vi "Photon-STR18_1_1.vi"() -> ()   [LabVIEW 2015]
uses:
  Menu.ctl
  <vilib>/Utility/file.llb/Write Delimited Spreadsheet (DBL).vi
panel:
  out "sizeA":i32
  out "mean 2":ext format="%0.2f"
  out "max index(es)":i32
  out "max value":u16
  out "Waveform Graph 5":dbl[][](graph)
  out "Waveform Graph 4":u8[][](graph)
  out "Size B":i32
  out "Size A":i32
  out "Waveform Graph 3":sgl[][](graph)
  out "8bits?":bool
  out "Waveform Graph 2":dbl[][](graph)
  out "P 2":i32=64
  out "m 2":i32=2
  in  "P":i32=64
  out "Numeric":i32
  out "sum A":dbl format="%#_10g"
  out "sum B":dbl format="%#_10g"
  out "Correlacion":cluster{ext[], ext[]}(graph)
  out "# of Channels":i32
  out "Duration":sgl
  in  "m":i32=2
  out "time":ext[](array[numeric])
  out "corr":ext[](array[numeric])
  out "d*(k)":dbl[][](array[numeric])
  out "Structura":cluster{ext[], ext[]}(graph)
  out "g(k) lineal":ext[](array[numeric])
  out "millisecond timer value":u32
  in  "Sample  time (a.u.)":sgl=1000.0
  out "segmentation ChA":sgl[](array[numeric])
  out "tau":dbl[](array[numeric]) format="%#_12g"
  out "Duration A [s]":dbl
  out "tau 3":dbl[](array[numeric]) format="%#_10g"
  out "Segmentation ChB 2":sgl[](array[numeric])
  out "Duration B [s] 2":dbl
  out "tamaño B 2":i32
  out "tau 2":dbl[](array[numeric]) format="%#_10g"
  out "Segmentation ChB":sgl[](array[numeric])
  out "Duration B [s]":dbl
  out "Size B":i32
  out "mean":dbl format="%0.2f"
  out "Size A":i32
  out "size(s) 2":i32
  out "time out":dbl[](array[numeric]) format="%#_10g"
  out "Max photon CHA 3":i32
  out "Numeric 2":i32
  out "size(s)":i32
  out "size(s) 7":i32
  out "Max photon CHA 4":i32
  out "size(s) 4":i32
  out "Max photon CHA 6":i32
  out "Numeric 3":i32
  out "size(s) 5":i32
  out "size(s) 6":i32
  out "Max photon CHA":i32
  out "Max photon CHA 2":i32
  out "element":sgl
  out "CHA":u8[](array[numeric])
  out "CHB":u8[](array[numeric])
  in  "Save Data":bool
  in  "Half data":bool
  in  "EXIT":bool
  in  "Open File":bool
  in  "Analysis":u16(ring) items=["Auto correlation A", "Auto correlation B", "Cross correlation AxB", "Cross correlation BxA"]
  in  "Data type":u16(ring) items=["Ascii", "Binary"]
  out "elapsed time in min":dbl
  out "Elapsed time (s)":dbl
  # "PhotonSTR-18"
  # "Parameters"
  # "Duration A"
  # "Total # of photons A"
  # "Channel A"
  # "Duration B"
  # "Total # of photons B"
  # "Operation Mode"
  # "Channel B"
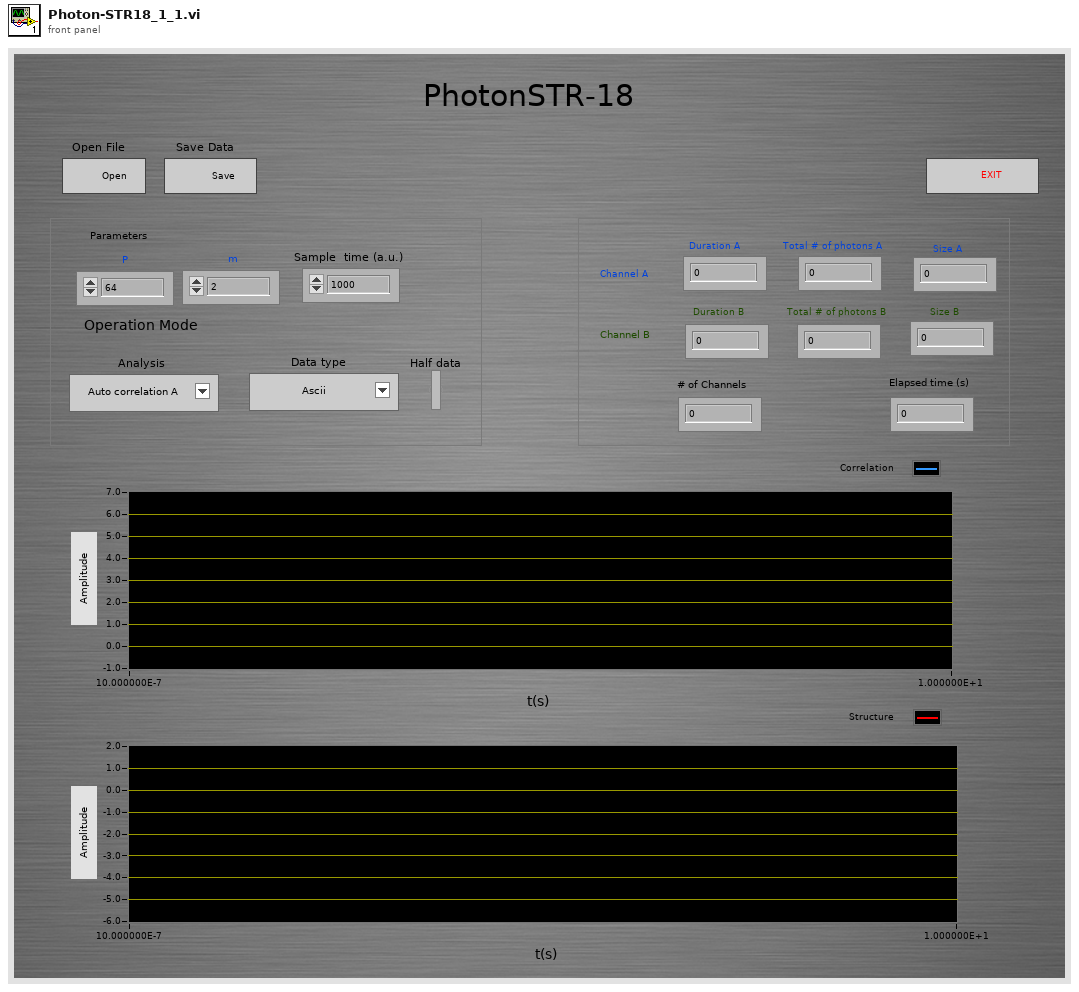
[diagram p1: front panel]
types:
  T1 = typedef "Menu.ctl" = enum16{"Init", "user action", "Load file", "Select range", "Process Photons(t)", "Process Segmentation", "Process Correlation ", "Save data", "Stop"}
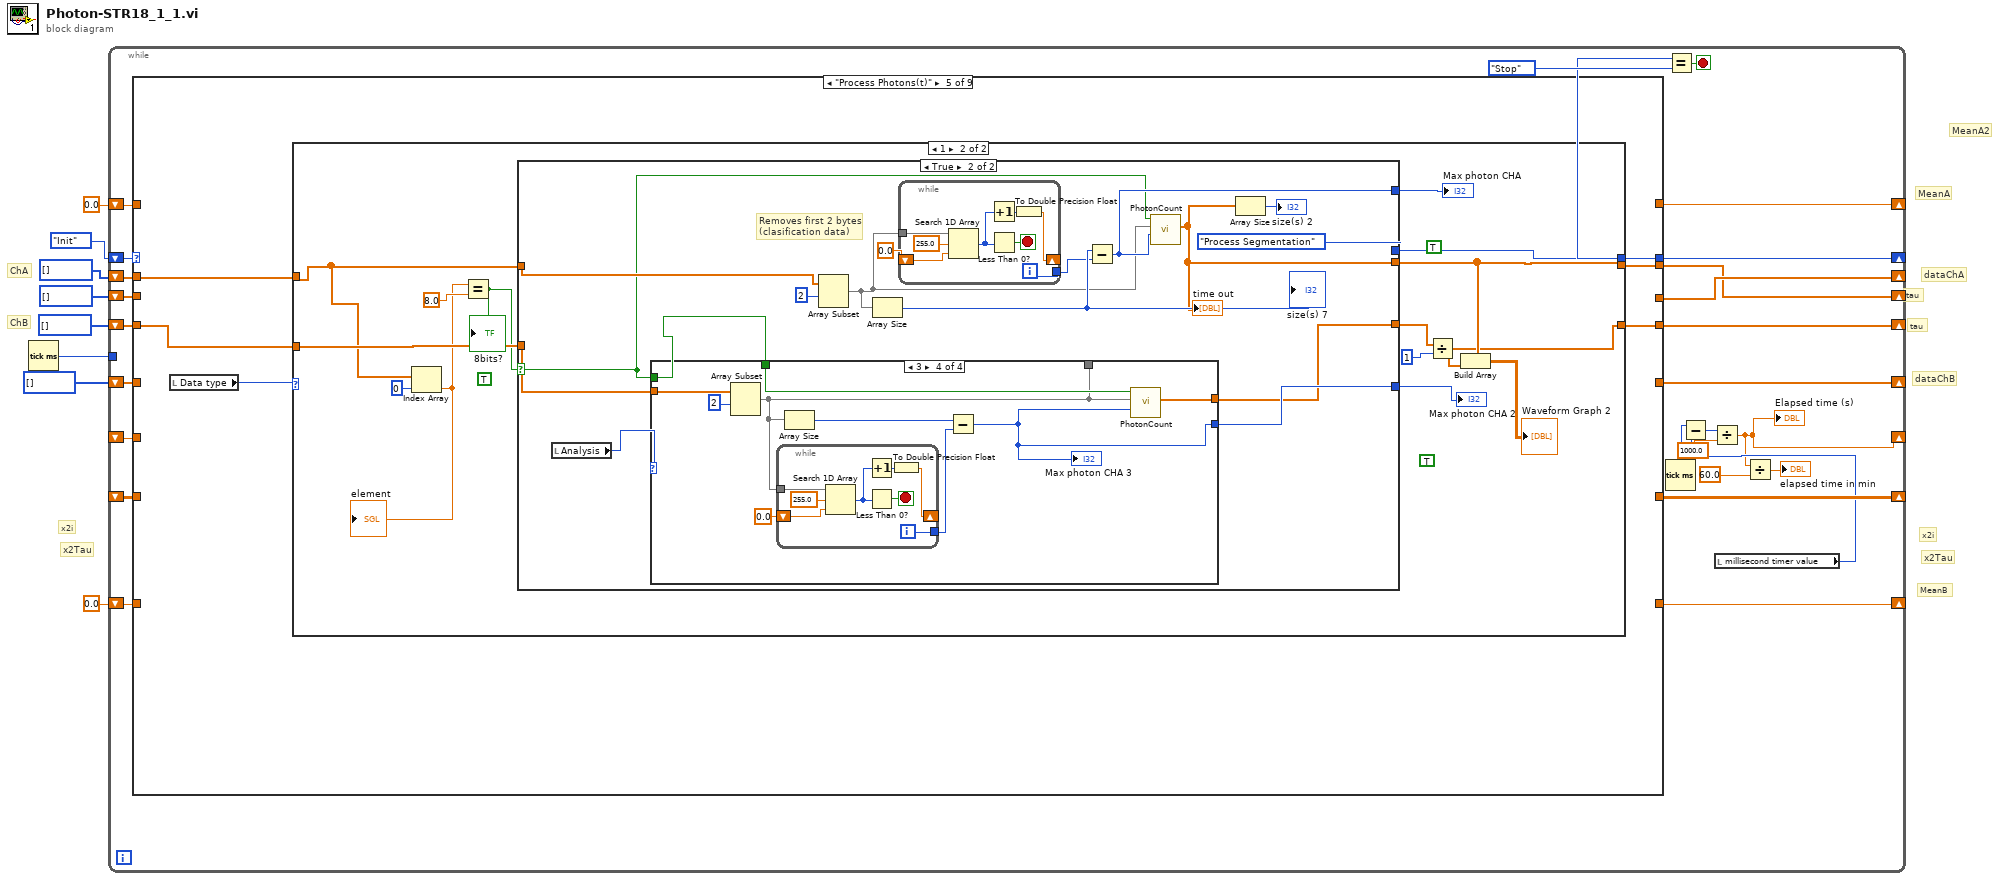
[diagram p0: block diagram]
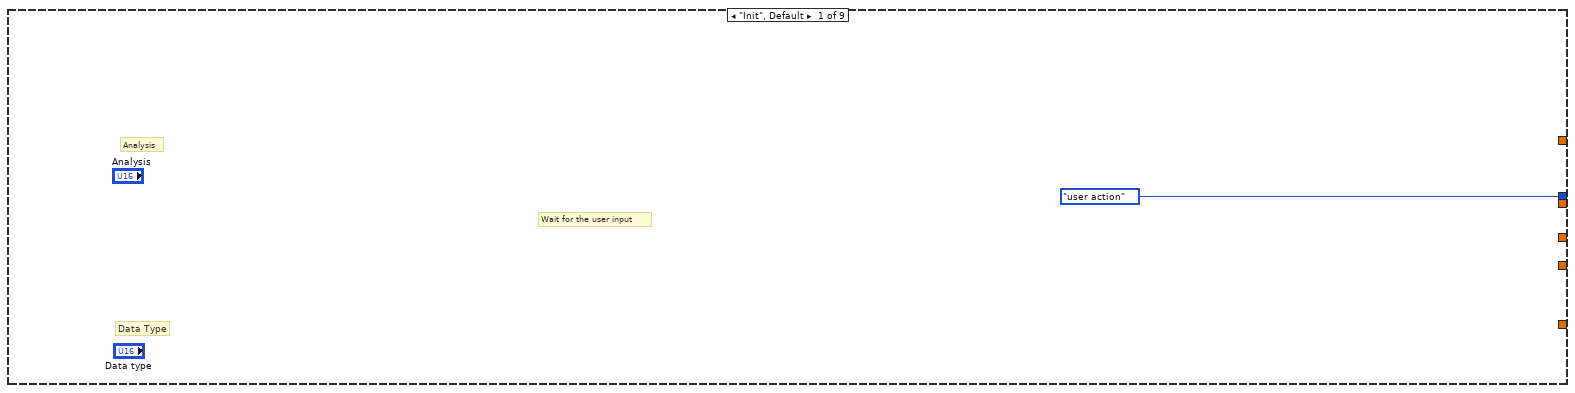
[diagram p2: hidden frame]
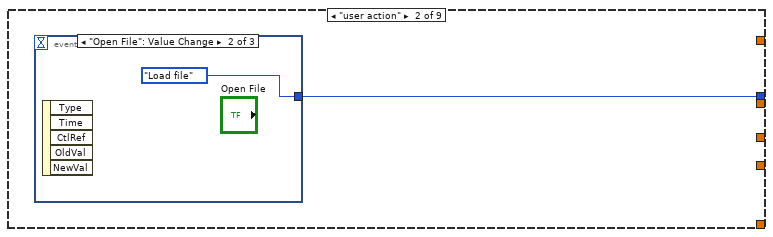
[diagram p3: hidden frame]
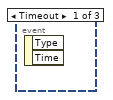
[diagram p4: hidden frame]
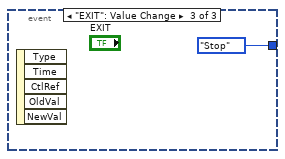
[diagram p5: hidden frame]
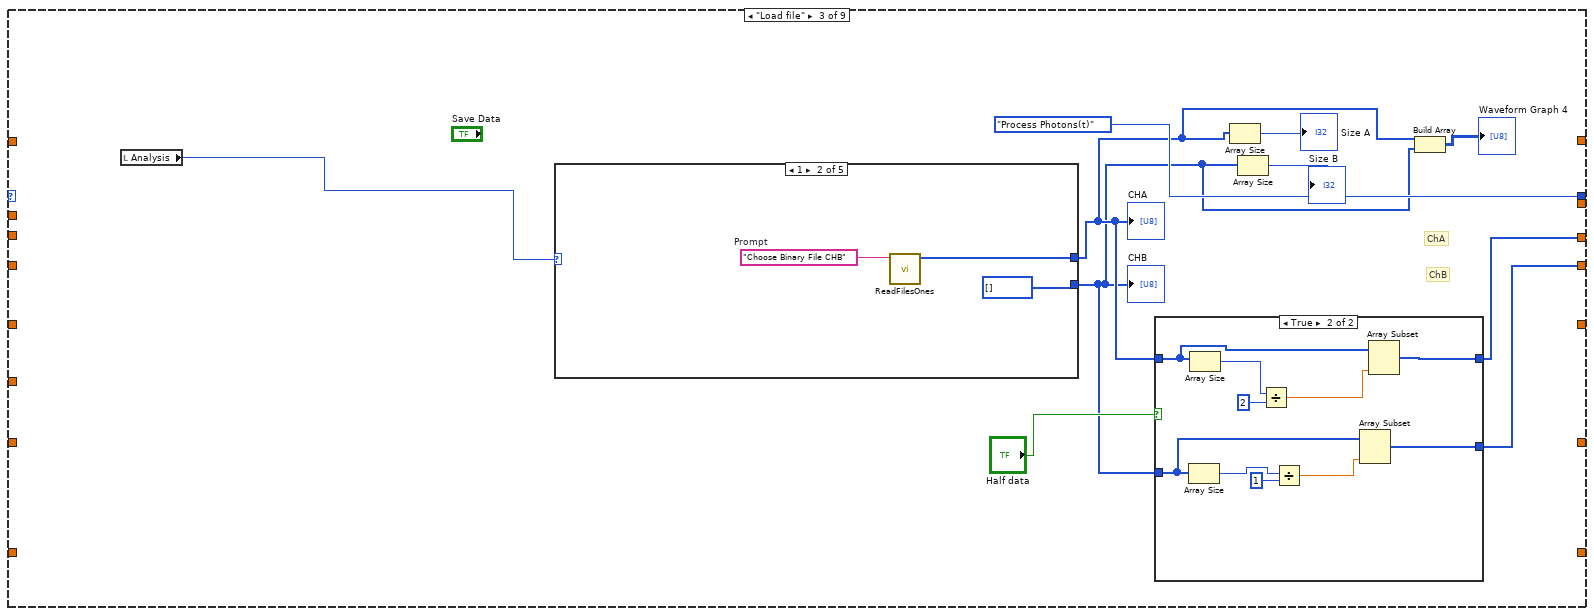
[diagram p6: hidden frame]
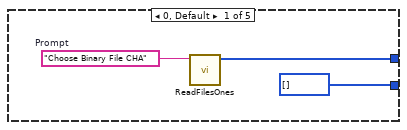
[diagram p8: hidden frame]
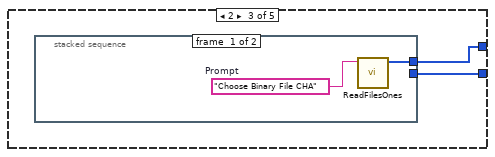
[diagram p9: hidden frame]
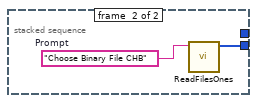
[diagram p10: hidden frame]
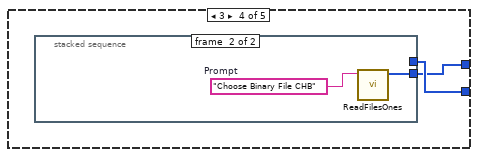
[diagram p11: hidden frame]
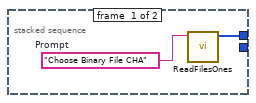
[diagram p12: hidden frame]
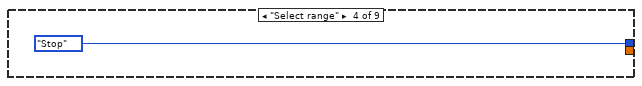
[diagram p14: hidden frame]
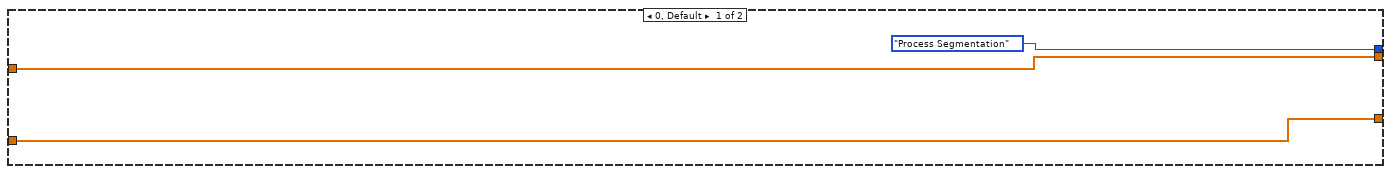
[diagram p15: hidden frame]
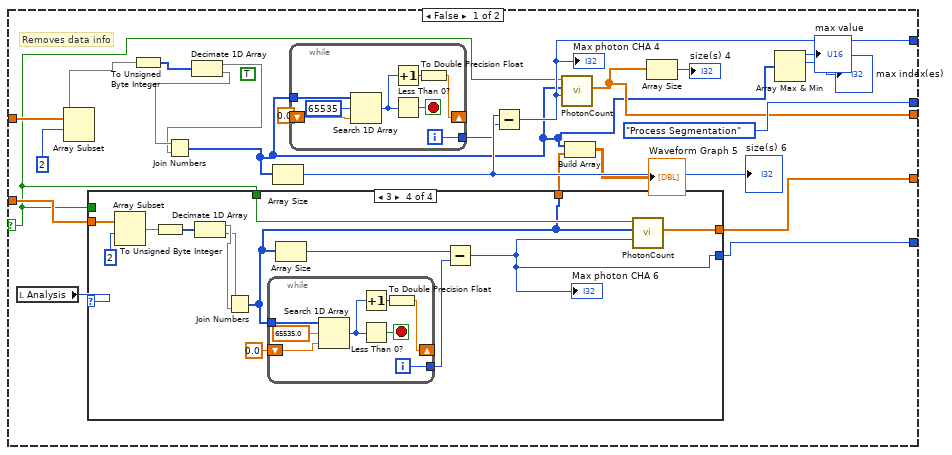
[diagram p16: hidden frame]
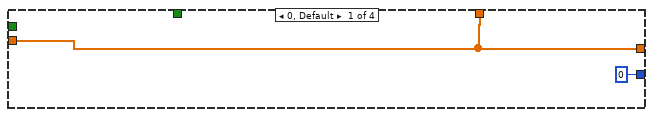
[diagram p17: hidden frame]
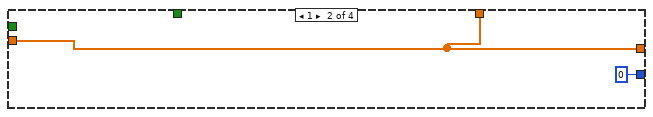
[diagram p18: hidden frame]
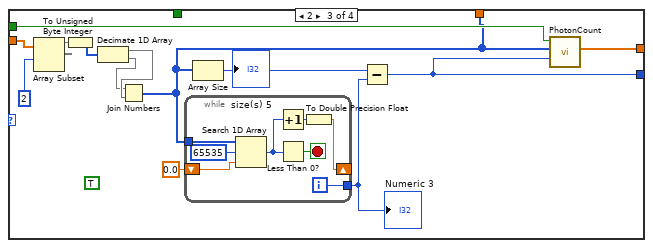
[diagram p19: hidden frame]
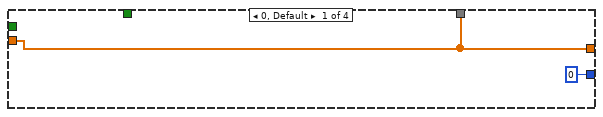
[diagram p20: hidden frame]
diagram:
  # "x2Tau"
  # "x2i"
  # "x2Tau"
  # "x2i"
  # "MeanA2"
  # "MeanB"
  # "MeanA"
  # "tau"
  # "tau"
  # "ChB"
  # "dataChB"
  # "dataChA"
  # "ChA"
  n1 = Tick Count (ms)() -> (millisecond timer value=w5:u32)
  n2 = while {
    shift-right: [w32] -> _
    shift-left: Menu."Init" ("Menu") -> [w34]
    shift-right: [w30] -> _
    shift-left: u32[] [] ("Photon trace A") -> [w29]
    shift-right: [w28] -> _
    shift-left: u32[] [] ("Photon trace A") -> [w27]
    shift-right: [w16] -> _
    shift-left: _ -> [w26]
    tunnel: w5 -> [_]
    shift-right: [w20] -> _
    shift-left: u32[] [] ("Photon trace A") -> [w19]
    shift-right: [w18] -> _
    shift-left: u32[] [] ("Photon trace A") -> [w17]
    shift-right: [w13] -> _
    shift-left: _ -> [w15]
    shift-right: [w12] -> _
    shift-left: 0.0 ("mean") -> [w10]
    shift-right: [w11] -> _
    shift-left: 0.0 ("mean") -> [w9]
    stop <- w31 stop-if-true
    n3 = case shown="\"Process Photons(t)\"" w34 {
      tunnel: [Menu."user action" ("Menu") w36 Menu."Process Photons(t)" ("Menu") Menu."Stop" ("Menu") w85 Menu."Process Correlation " ("Menu") Menu."Save data" ("Menu") Menu."Stop" ("Menu") Menu."Stop" ("Menu")] -> w32
      tunnel: [_ _ w44 _ _ w244 _ _ _] -> w30
      tunnel: w29 -> [_ _ _ _ w84 _ w336 _ _]
      tunnel: [_ _ _ _ w81 w252 _ _ _] -> w28
      tunnel: w27 -> [_ _ _ _ _ w261 w340 _ _]
      tunnel: [_ _ _ _ _ _ w369 _ _] -> w16
      tunnel: w26 -> [_ _ _ _ _ _ _ w435 _]
      tunnel: [_ _ w45 _ w82 w250 _ _ _] -> w20
      tunnel: w19 -> [_ _ _ _ w83 w262 _ _ _]
      tunnel: [_ _ _ _ _ w246 _ _ _] -> w18
      tunnel: w17 -> [_ _ _ _ _ _ w335 _ _]
      tunnel: w15 -> [_ _ _ _ _ _ _ _ _]
      tunnel: [_ _ _ _ _ w241 _ _ _] -> w12
      tunnel: [_ _ _ _ _ w248 _ _ _] -> w11
      tunnel: w10 -> [_ _ _ _ _ _ w368 _ _]
      tunnel: w9 -> [_ _ _ _ _ _ w367 _ _]
      frame "Init", Default {
        # "Data Type"
        # "Analysis"
        # "Wait for the user input"
      }
      frame "user action" {
        n4 = event shown="[1] \"Open File\": Value Change" {
          selector: _ -> [_ _ _]
          dyn-events: _ -> [_ _ _]
          timeout: _ -> [_ _ _]
          tunnel: [_ Menu."Load file" ("Menu") Menu."Stop" ("Menu")] -> w36
          event Timeout {
            n5 = event-data() -> ()  [unwired: 1 in, 2 out]
          }
          event "Open File": Value Change {
            n6 = event-data() -> ()  [unwired: 1 in, 5 out]
          }
          event "EXIT": Value Change {
            n7 = event-data() -> ()  [unwired: 1 in, 5 out]
          }
        }
      }
      frame "Load file" {
        # "ChB"
        # "ChA"
        n8 = local read "Analysis"() -> (w47:u16)
        n9 = case shown="1" w47 {
          tunnel: [w62 w65 w68 w73 _] -> w41
          tunnel: [u8[] [] u8[] [] w67 w74 _] -> w40
          frame 0, Default {
            w63 = "Choose Binary File CHA"  # Prompt
            n10 = call "ReadFilesOnes.vi"("prompt"=w63) -> ("Data"=w62:u8[])  [unwired: 8 in, 2 out]
          }
          frame 1 {
            w66 = "Choose Binary File CHB"  # Prompt
            n11 = call "ReadFilesOnes.vi"("prompt"=w66) -> ("Data"=w65:u8[])  [unwired: 8 in, 2 out]
          }
          frame 2 {
            n12 = stacked-sequence {
              tunnel: [w69 _] -> w68
              tunnel: [_ w71] -> w67
              frame #0 {
                w70 = "Choose Binary File CHA"  # Prompt
                n13 = call "ReadFilesOnes.vi"("prompt"=w70) -> ("Data"=w69:u8[])  [unwired: 8 in, 2 out]
              }
              frame #1 {
                w72 = "Choose Binary File CHB"  # Prompt
                n14 = call "ReadFilesOnes.vi"("prompt"=w72) -> ("Data"=w71:u8[])  [unwired: 8 in, 2 out]
              }
            }
          }
          frame 3 {
            n15 = stacked-sequence {
              tunnel: [w75 _] -> w74
              tunnel: [_ w77] -> w73
              frame #0 {
                w76 = "Choose Binary File CHA"  # Prompt
                n16 = call "ReadFilesOnes.vi"("prompt"=w76) -> ("Data"=w75:u8[])  [unwired: 8 in, 2 out]
              }
              frame #1 {
                w78 = "Choose Binary File CHB"  # Prompt
                n17 = call "ReadFilesOnes.vi"("prompt"=w78) -> ("Data"=w77:u8[])  [unwired: 8 in, 2 out]
              }
            }
          }
          frame 4 {
          }
        }
        "CHA" <- w41
        "CHB" <- w40
        n18 = case shown="True" "Half data" {
          tunnel: w41 -> [w50 w60]
          tunnel: w40 -> [w49 w59]
          tunnel: [w50 w57] -> w44
          tunnel: [w49 w56] -> w45
          frame False {
          }
          frame True {
            n19 = Array Size(array=w59) -> (size(s)=w55:i32)
            n20 = Array Size(array=w60) -> (size(s)=w58:i32)
            n21 = Divide(x=w58, y=2) -> (x/y=w54:dbl)
            n22 = Divide(x=w55, y=1) -> (x/y=w53:dbl)
            n23 = Array Subset(array=w59, length=w53) -> (w56:u8[])  [unwired: 1 in]
            n24 = Array Subset(array=w60, length=w54) -> (w57:u8[])  [unwired: 1 in]
          }
        }
        n25 = Array Size(array=w41) -> (size(s)=→"Size A":i32)
        n26 = Array Size(array=w40) -> (size(s)=→"Size B":i32)
        n27 = Build Array(w41, w40) -> (→"Waveform Graph 4":u8[][])
      }
      frame "Select range" {
      }
      frame "Process Photons(t)" {
        n28 = local read "Data type"() -> (w80:u16)
        n29 = case shown="1" w80 {
          tunnel: [Menu."Process Segmentation" ("Menu") w101] -> w85
          tunnel: w84 -> [w87 w99]
          tunnel: w83 -> [w86 w102]
          tunnel: [w86 w89] -> w82
          tunnel: [w87 w93] -> w81
          frame 0, Default {
          }
          frame 1 {
            (unwired) TRUE ("transpose? (no:F)")
            (unwired) TRUE ("transpose? (no:F)")
            (unwired) TRUE
            n30 = Index Array(array=w99, index=0) -> (element=w97:sgl)
            "element" <- w97
            n31 = Equal?(x=w97, y=8.0) -> (x = y?=w94:bool)
            "8bits?" <- w94
            n32 = case shown="True" w94 {
              selector: w94 -> [w103 w181]
              tunnel: w102 -> [w115 w189]
              tunnel: [w120 w182] -> w91
              tunnel: [w116 w188] -> w93
              tunnel: [Menu."Process Segmentation" ("Menu") Menu."Process Segmentation" ("Menu")] -> w101
              tunnel: w99 -> [w113 w185]
              tunnel: [w117 w184] -> w96
              tunnel: [w118 w183] -> w95
              frame False {
                (unwired) TRUE ("transpose? (no:F)")
                # "Removes data info"
                n33 = local read "Analysis"() -> (w119:u16)
                n34 = Array Subset(array=w113, index=2) -> (w105:sgl[])  [unwired: 1 in]
                n35 = case shown="3" w119 {
                  tunnel: w115 -> [w126 w128 w135 w156]
                  tunnel: [w126 w128 w138 w159] -> w120
                  tunnel: [0 0 w137 w158] -> w118
                  tunnel: w103 -> [_ _ w136 _]
                  tunnel: w103 -> [_ _ _ w157]
                  tunnel: [w126 w128 w132 w153] -> w110
                  frame 0, Default {
                  }
                  frame 1 {
                  }
                  frame 2 {
                    (unwired) TRUE ("transpose? (no:F)")
                    n36 = Array Subset(array=w135, index=2) -> (w131:dbl[])  [unwired: 1 in]
                    n37 = To Unsigned Byte Integer(number=w131) -> (unsigned 8bit integer=w130:u8[])
                    n38 = Decimate 1D Array(w130) -> (w134:u8[], w133:u8[])
                    n39 = Join Numbers(hi=w133, lo=w134) -> ((hi.lo)=w132:u16[])
                    n40 = while {
                      tunnel: w132 -> [w150]
                      shift-right: [w143] -> _
                      shift-left: 0.0 ("element") -> [w148]
                      tunnel: [w146] -> w139
                      i -> [w146]
                      stop <- w147 stop-if-true
                      n41 = Search 1D Array(1D array=w150, element=u16 65535, start index (0)=w148) -> (index of element=w145:i32)
                      n42 = Increment(x=w145) -> (x+1=w144:i32)
                      n43 = Less Than 0?(x=w145) -> (x < 0?=w147:bool)
                      n44 = To Double Precision Float(number=w144) -> (double precision float=w143:dbl)
                    }
                    "Numeric 3" <- w139
                    n45 = Array Size(array=w132) -> (size(s)=w140:i32)
                    "size(s) 5" <- w140
                    n46 = Subtract(x=w140, y=w139) -> (x-y=w137:i32)
                    n47 = call "PhotonCount.vi"("# Photons"=w137, "Data in"=w132, "Boolean"=w136) -> ("time out"=w138:dbl[])  [unwired: 8 in]
                  }
                  frame 3 {
                    n48 = Array Subset(array=w156, index=2) -> (w152:dbl[])  [unwired: 1 in]
                    n49 = To Unsigned Byte Integer(number=w152) -> (unsigned 8bit integer=w151:u8[])
                    n50 = Decimate 1D Array(w151) -> (w155:u8[], w154:u8[])
                    n51 = Join Numbers(hi=w154, lo=w155) -> ((hi.lo)=w153:u16[])
                    n52 = while {
                      tunnel: w153 -> [w171]
                      shift-right: [w164] -> _
                      shift-left: 0.0 ("element") -> [w169]
                      tunnel: [w167] -> w160
                      i -> [w167]
                      stop <- w168 stop-if-true
                      n53 = Search 1D Array(1D array=w171, element=sgl 65535.0, start index (0)=w169) -> (index of element=w166:i32)
                      n54 = Increment(x=w166) -> (x+1=w165:i32)
                      n55 = Less Than 0?(x=w166) -> (x < 0?=w168:bool)
                      n56 = To Double Precision Float(number=w165) -> (double precision float=w164:dbl)
                    }
                    n57 = Array Size(array=w153) -> (size(s)=w161:i32)
                    n58 = Subtract(x=w161, y=w160) -> (x-y=w158:i32)
                    "Max photon CHA 6" <- w158
                    n59 = call "PhotonCount.vi"("# Photons"=w158, "Data in"=w153, "Boolean"=w157) -> ("time out"=w159:dbl[])  [unwired: 8 in]
                  }
                }
                n60 = To Unsigned Byte Integer(number=w105) -> (unsigned 8bit integer=w104:u8[])
                n61 = Decimate 1D Array(w104) -> (w111:u8[], w112:u8[])
                n62 = Join Numbers(hi=w112, lo=w111) -> ((hi.lo)=w108:u16[])
                n63 = Array Size(array=w108) -> (size(s)=w124:i32)
                "size(s) 6" <- w124
                n64 = while {
                  tunnel: w108 -> [w179]
                  shift-right: [w173] -> _
                  shift-left: 0.0 ("element") -> [w177]
                  tunnel: [w172] -> w123
                  i -> [w172]
                  stop <- w176 stop-if-true
                  n65 = Search 1D Array(1D array=w179, element=u16 65535, start index (0)=w177) -> (index of element=w175:i32)
                  n66 = Increment(x=w175) -> (x+1=w174:i32)
                  n67 = Less Than 0?(x=w175) -> (x < 0?=w176:bool)
                  n68 = To Double Precision Float(number=w174) -> (double precision float=w173:dbl)
                }
                n69 = Subtract(x=w124, y=w123) -> (x-y=w117:i32)
                "Max photon CHA 4" <- w117
                n70 = call "PhotonCount.vi"("# Photons"=w117, "Data in"=w108, "Boolean"=w103) -> ("time out"=w116:dbl[])  [unwired: 8 in]
                n71 = Build Array(w108, w110) -> (→"Waveform Graph 5":dbl[][])
                n72 = Array Size(array=w116) -> (size(s)=→"size(s) 4":i32)
                n73 = Array Max & Min(array=w108) -> (max value=→"max value":u16, max index (indices)=→"max index(es)":i32)  [unwired: 2 out]
              }
              frame True {
                # "Removes first 2 bytes\n(clasification data)"
                n74 = local read "Analysis"() -> (w186:u16)
                n75 = case shown="3" w186 {
                  tunnel: w189 -> [w195 w197 w206 w220]
                  tunnel: [w195 w197 w202 w219] -> w182
                  tunnel: [0 0 w201 w218] -> w183
                  tunnel: w181 -> [_ _ w200 _]
                  tunnel: w181 -> [_ _ _ w217]
                  tunnel: [w195 w197 w199 w216] -> _
                  frame 0, Default {
                  }
                  frame 1 {
                  }
                  frame 2 {
                    n76 = Array Subset(array=w206, index=2) -> (w199:dbl[])  [unwired: 1 in]
                    n77 = while {
                      tunnel: w199 -> [w215]
                      shift-right: [w208] -> _
                      shift-left: 0.0 ("element") -> [w213]
                      tunnel: [w211] -> w203
                      i -> [w211]
                      stop <- w212 stop-if-true
                      n78 = Search 1D Array(1D array=w215, element=sgl 255.0, start index (0)=w213) -> (index of element=w210:i32)
                      n79 = Increment(x=w210) -> (x+1=w209:i32)
                      n80 = Less Than 0?(x=w210) -> (x < 0?=w212:bool)
                      n81 = To Double Precision Float(number=w209) -> (double precision float=w208:dbl)
                    }
                    "Numeric 2" <- w203
                    n82 = Array Size(array=w199) -> (size(s)=w204:i32)
                    "size(s)" <- w204
                    n83 = Subtract(x=w204, y=w203) -> (x-y=w201:i32)
                    n84 = call "PhotonCount.vi"("# Photons"=w201, "Data in"=w199, "Boolean"=w200) -> ("time out"=w202:dbl[])  [unwired: 8 in]
                  }
                  frame 3 {
                    n85 = Array Subset(array=w220, index=2) -> (w216:dbl[])  [unwired: 1 in]
                    n86 = while {
                      tunnel: w216 -> [w232]
                      shift-right: [w225] -> _
                      shift-left: 0.0 ("element") -> [w230]
                      tunnel: [w228] -> w221
                      i -> [w228]
                      stop <- w229 stop-if-true
                      n87 = Search 1D Array(1D array=w232, element=sgl 255.0, start index (0)=w230) -> (index of element=w227:i32)
                      n88 = Increment(x=w227) -> (x+1=w226:i32)
                      n89 = Less Than 0?(x=w227) -> (x < 0?=w229:bool)
                      n90 = To Double Precision Float(number=w226) -> (double precision float=w225:dbl)
                    }
                    n91 = Array Size(array=w216) -> (size(s)=w222:i32)
                    n92 = Subtract(x=w222, y=w221) -> (x-y=w218:i32)
                    "Max photon CHA 3" <- w218
                    n93 = call "PhotonCount.vi"("# Photons"=w218, "Data in"=w216, "Boolean"=w217) -> ("time out"=w219:dbl[])  [unwired: 8 in]
                  }
                }
                n94 = Array Subset(array=w185, index=2) -> (w180:sgl[])  [unwired: 1 in]
                n95 = Array Size(array=w180) -> (size(s)=w192:i32)
                "size(s) 7" <- w192
                n96 = while {
                  tunnel: w180 -> [w240]
                  shift-right: [w233] -> _
                  shift-left: 0.0 ("element") -> [w238]
                  tunnel: [w236] -> w191
                  i -> [w236]
                  stop <- w237 stop-if-true
                  n97 = Search 1D Array(1D array=w240, element=sgl 255.0, start index (0)=w238) -> (index of element=w235:i32)
                  n98 = Increment(x=w235) -> (x+1=w234:i32)
                  n99 = Less Than 0?(x=w235) -> (x < 0?=w237:bool)
                  n100 = To Double Precision Float(number=w234) -> (double precision float=w233:dbl)
                }
                n101 = Subtract(x=w192, y=w191) -> (x-y=w184:i32)
                n102 = call "PhotonCount.vi"("# Photons"=w184, "Data in"=w180, "Boolean"=w181) -> ("time out"=w188:dbl[])  [unwired: 8 in]
                "time out" <- w188
                n103 = Array Size(array=w188) -> (size(s)=→"size(s) 2":i32)
              }
            }
            "Max photon CHA" <- w96
            "Max photon CHA 2" <- w95
            n104 = Divide(x=w91, y=1 ("Data Type (DBL)")) -> (x/y=w89:dbl[])
            n105 = Build Array(w93, w89) -> (→"Waveform Graph 2":dbl[][])
          }
        }
      }
      frame "Process Segmentation" {
        w255 = 60000000.0 ("x")
        # "Estima la segmentacion de datos"
        n106 = local read "Analysis"() -> (w245:u16)
        n107 = call "Segmentation.vi"("sample time"="Sample  time (a.u.)", "relative time"=w261) -> ("Segmentation"=w242:sgl[], "mean"=w241:dbl, "tau"=w243:dbl[])  [unwired: 7 in]
        "segmentation ChA" <- w242
        "tau" <- w243
        "mean 2" <- w241
        n108 = Array Size(array=w242) -> (size(s)=w247:i32)
        "Size A" <- w247
        "sizeA" <- w247
        n109 = case shown="2" w245 {
          tunnel: w262 -> [w268 w272 w284 w291]
          tunnel: "Sample  time (a.u.)" -> [_ _ w283 w290]
          tunnel: w255 -> [_ _ w278 w289]
          tunnel: [w266 w271 w276 w287] -> w253
          tunnel: [w268 w272 w277 w288] -> w251
          tunnel: [sgl[] [] sgl[] [] w274 w285] -> w249
          tunnel: w247 -> [w266 w271 _ _]
          tunnel: [0.0 ("mean") 0.0 ("mean") w275 w286] -> w248
          tunnel: w242 -> [w264 w269 _ _]
          tunnel: [w264 w269 w274 w285] -> _
          frame 0, Default {
          }
          frame 1 {
          }
          frame 2 {
            n110 = call "Segmentation.vi"("sample time"=w283, "relative time"=w284) -> ("Segmentation"=w274:sgl[], "mean"=w275:dbl, "tau"=w277:dbl[])  [unwired: 7 in]
            "tau 2" <- w277
            "Segmentation ChB" <- w274
            "mean" <- w275
            n111 = Array Size(array=w277) -> (size(s)=w276:i32)
            "Size B" <- w276
            n112 = Decrement(x=w276) -> (x-1=w282:i32)
            n113 = Index Array(array=w277, index=w282) -> (element=w281:dbl)
            n114 = Reciprocal(x=w278) -> (1/x=w280:dbl)
            n115 = Multiply(x=w281, y=w280) -> (x*y=→"Duration B [s]":dbl)
          }
          frame 3 {
            n116 = call "Segmentation.vi"("sample time"=w290, "relative time"=w291) -> ("Segmentation"=w285:sgl[], "mean"=w286:dbl, "tau"=w288:dbl[])  [unwired: 7 in]
            "tau 3" <- w288
            "Segmentation ChB 2" <- w285
            n117 = Array Size(array=w288) -> (size(s)=w287:i32)
            "tamaño B 2" <- w287
            n118 = Decrement(x=w287) -> (x-1=w295:i32)
            n119 = Index Array(array=w288, index=w295) -> (element=w294:dbl)
            n120 = Reciprocal(x=w289) -> (1/x=w293:dbl)
            n121 = Multiply(x=w294, y=w293) -> (x*y=→"Duration B [s] 2":dbl)
          }
        }
        n122 = Decrement(x=w247) -> (x-1=w259:i32)
        n123 = Index Array(array=w243, index=w259) -> (element=w256:dbl)
        n124 = Reciprocal(x=w255) -> (1/x=w258:dbl)
        n125 = Multiply(x=w256, y=w258) -> (x*y=→"Duration A [s]":dbl)
        n126 = Equal?(x=w247, y=w253) -> (x = y?=w254:bool)
        n127 = case shown="False" w254 {
          tunnel: w243 -> [w304 w324]
          tunnel: w242 -> [w303 w323]
          tunnel: w251 -> [w300 w326]
          tunnel: w249 -> [w301 w325]
          tunnel: w247 -> [w307 _]
          tunnel: w253 -> [w308 _]
          tunnel: [w299 w324] -> w252
          tunnel: [w298 w323] -> w244
          tunnel: [w297 w326] -> w250
          tunnel: [w296 w325] -> w246
          frame False {
            # "ChA>ChB"
            n128 = Greater?(x=w307, y=w308) -> (0:w305:bool)
            n129 = Subtract(x=w308, y=w307) -> (x-y=w306:i32)
            n130 = Absolute Value(x=w306) -> (abs(x)=w302:i32)
            n131 = case shown="False" w305 {
              tunnel: w304 -> [w310 w322]
              tunnel: w303 -> [w309 w321]
              tunnel: w302 -> [w315 w320]
              tunnel: [w310 w319] -> w299
              tunnel: [w309 w318] -> w298
              tunnel: w301 -> [w313 w316]
              tunnel: w300 -> [w314 w317]
              tunnel: [w311 w317] -> w297
              tunnel: [w312 w316] -> w296
              frame False {
                n132 = Delete From Array(array=w314, length=w315) -> (array with subset deleted=w311:dbl[])  [unwired: 1 in, 1 out]
                n133 = Delete From Array(array=w313, length=w315) -> (array with subset deleted=w312:sgl[])  [unwired: 1 in, 1 out]
              }
              frame True {
                n134 = Delete From Array(array=w322, length=w320) -> (array with subset deleted=w319:dbl[])  [unwired: 1 in, 1 out]
                n135 = Delete From Array(array=w321, length=w320) -> (array with subset deleted=w318:sgl[])  [unwired: 1 in, 1 out]
              }
            }
          }
          frame True {
          }
        }
      }
      frame "Process Correlation " {
        (unwired) 1.0 ("y")
        # "Calcula correlacion"
        # "g(k)=[G(k)-n0AnkB]/(n0AnkB))"
        # "Normalize"
        # "Compara que el tamaño\nde segmentation sea multiplo de m"
        n136 = Divide(x=w335, y=2 ("lower limit")) -> (x/y=w343:sgl[])
        n137 = Build Array(w336, w343) -> (→"Waveform Graph 3":sgl[][])
        n138 = To Double Precision Float(number=w335) -> (double precision float=w356:dbl[])
        n139 = To Double Precision Float(number=w336) -> (double precision float=w357:dbl[])
        n140 = while {
          tunnel: [w397] -> w328 mode=indexing
          shift-right: [w393] -> _
          shift-left: w357 -> [w390]
          tunnel: "m" -> [w387]
          tunnel: "P" -> [w388]
          tunnel: [w395] -> w337 mode=indexing
          shift-right: [w382] -> _
          shift-left: w356 -> [w389]
          tunnel: w368 -> [w386]
          tunnel: w367 -> [w385]
          tunnel: [w384] -> w331
          tunnel: [w383] -> w334
          tunnel: [w381] -> w327
          i -> [w394]
          stop <- w398 stop-if-true
          n141 = local read "Analysis"() -> (w381:u16)
          n142 = case shown="1" w381 {
            tunnel: w390 -> [w424 w426 w430 w434]
            tunnel: [w424 w426 w430 w434] -> w380
            tunnel: [w424 w426 w429 w433] -> w379
            tunnel: w389 -> [_ _ w429 w433]
            tunnel: w386 -> [w423 w425 w428 w432]
            tunnel: w385 -> [_ _ w427 w431]
            tunnel: [w423 w425 w428 w432] -> w384
            tunnel: [w423 w425 w427 w431] -> w383
            frame 0, Default {
            }
            frame 1 {
            }
            frame 2 {
            }
            frame 3 {
            }
          }
          n143 = case shown="0, Default" w381 {
            tunnel: [w403 w408 w415 w422] -> w397
            tunnel: w388 -> [w401 w406 w414 w417]
            tunnel: w387 -> [w400 w405 w413 w416]
            tunnel: [w399 w404 w412 w421] -> w393
            tunnel: [w399 w404 w411 w420] -> w382
            tunnel: w379 -> [_ _ w410 w418]
            tunnel: w380 -> [w402 w407 w409 w419]
            frame 0, Default {
              n144 = call "Auto_corr.vi"("m"=w400, "P"=w401, "input A"=w402) -> ("Sn"=w399:dbl[], "Acc"=w403:dbl[])  [unwired: 7 in]
            }
            frame 1 {
              n145 = call "Auto_corr.vi"("m"=w405, "P"=w406, "input A"=w407) -> ("Sn"=w404:dbl[], "Acc"=w408:dbl[])  [unwired: 7 in]
            }
            frame 2 {
              n146 = call "Cross_corr.vi"("m"=w413, "P"=w414, "input B"=w410, "input A"=w409) -> ("Sn A"=w412:dbl[], "Acc"=w415:dbl[], "Sn B"=w411:dbl[])  [unwired: 5 in]
            }
            frame 3 {
              n147 = call "Cross_corr.vi"("m"=w416, "P"=w417, "input B"=w418, "input A"=w419) -> ("Sn A"=w421:dbl[], "Acc"=w422:dbl[], "Sn B"=w420:dbl[])  [unwired: 5 in]
            }
          }
          n148 = Array Size(array=w393) -> (size(s)=w396:i32)
          n149 = Add Array Elements(numeric array=w393) -> (sum=→"sum A":dbl)
          n150 = Add Array Elements(numeric array=w382) -> (sum=→"sum B":dbl)
          n151 = Less Or Equal?(x=w396, y=w387) -> (x <= y?=w398:bool)
          n152 = Array Size(array=w380) -> (size(s)=w395:i32)
          "Numeric" <- w394
        }
        n153 = call "Normalizer.vi"("Acc"=w328, "m"="m", "p"="P", "Tamaño Sn"=w337, "Analysis 2"=w327, "AvgA"=w331, "DataA"=w336, "AvgB"=w334, "DataB"=w335) -> ("g(k)"=w333:dbl[][], "s(k)"=w330:dbl[][])  [unwired: 9 in]
        "d*(k)" <- w330
        n154 = Array Size(array=w328) -> (size(s)=w329:i32[])
        n155 = call "Data_select.vi"("m"="m", "P"="P", "d(k) in"=w330, "g(k) in"=w333) -> ("d(k) lineal"=w352:ext[], "g(k) lineal"=w342:ext[])  [unwired: 6 in]
        "g(k) lineal" <- w342
        n156 = Tick Count (ms)() -> (millisecond timer value=→"millisecond timer value":u32)
        n157 = Index Array(array=w329, index=0) -> (element=w358:i32)
        n158 = case shown="True" TRUE {
          tunnel: w342 -> [w372 w374]
          tunnel: [w371 w373] -> w349
          frame False {
            n159 = Array Size(array=w372) -> (size(s)=w371:i32)
          }
          frame True {
            n160 = while {
              tunnel: w374 -> [w378] mode=indexing
              tunnel: [w375] -> w373
              i -> [w376]
              stop <- w377 stop-if-true
              n161 = Not A Number/Path/Refnum?(number/path/refnum=w378) -> (NaN/Path/Refnum?=w377:bool)
              n162 = To Double Precision Float(number=w376) -> (double precision float=w375:dbl)
            }
          }
        }
        n163 = call "multi-tau_time.vi"("tau"=w340, "m"="m", "P"="P", "No. of shift registers"=w358) -> ("time multi-tau"=w341:ext[])  [unwired: 7 in]
        n164 = Divide(x=w341, y=60000000.0) -> (x/y=w332:ext[])
        n165 = Array Subset(array=w352, index=0) -> (w348:ext[])  [unwired: 1 in]
        n166 = Array Subset(array=w342, index=0, length=w349) -> (w355:ext[])
        "corr" <- w355
        n167 = Array Subset(array=w332, index=0, length=w349) -> (w350:ext[])
        "time" <- w350
        n168 = Array Size(array=w355) -> (size(s)=→"# of Channels":i32)
        n169 = Bundle(w350, w355) -> (→"Correlacion":cluster{ext[], ext[]})  [unwired: 1 in]
        n170 = Bundle(w350, w348) -> (→"Structura":cluster{ext[], ext[]})  [unwired: 1 in]
        n171 = Array Size(array=w350) -> (size(s)=w364:i32)
        n172 = Build Array(w350, w355, w348) -> (w369:ext[][])
        n173 = Decrement(x=w364) -> (x-1=w363:i32)
        n174 = Index Array(array=w350, index=w363) -> (element=→"Duration":ext)
        "m 2" <- "m"
        "P 2" <- "P"
      }
      frame "Save data" {
        # "Save data"
        n175 = Two Button Dialog(message="Do you want to save the data?", 1:"No" ("F button name (\"Cancel\")"), 2:"Yes" ("T button name (\"OK\")")) -> (T button?=w436:bool)
        n176 = case shown="True" w436 {
          tunnel: w435 -> [_ w443]
          frame False {
          }
          frame True {
            n177 = Transpose 2D Array(2D array=w443) -> (transposed array=w441:ext[][])
            n178 = call-poly <vilib>:"Write Delimited Spreadsheet.vi"("format (%.3f)"="%.6e", "2D data"=w441) -> ()  [unwired: 12 in, 2 out]
          }
        }
      }
      frame "Stop" {
        # "Registry cleanse"
      }
    }
    n179 = Tick Count (ms)() -> (millisecond timer value=w23:u32)
    n180 = Equal?(x=w32, y=Menu."Stop" ("Menu")) -> (x = y?=w31:bool)
    n181 = local read "millisecond timer value"() -> (w14:u32)
    n182 = Subtract(x=w23, y=w14) -> (x-y=w25:u32)
    n183 = Divide(x=w25, y=1000.0) -> (x/y=w13:dbl)
    "Elapsed time (s)" <- w13
    n184 = Divide(x=w13, y=60.0) -> (x/y=→"elapsed time in min":dbl)
  }
